vi "DefensePsSkill.vi"(9 "Game in":refnum<class "Game.lvclass">, 10 "Robot":refnum<class "Robot.lvclass">, 11 "DefensePsSkill in":refnum<class "DefensePsSkill.lvclass">) -> (2 "Robot out":refnum<class "Robot.lvclass">, 3 "DefensePsSkill out":refnum<class "DefensePsSkill.lvclass">)   [LabVIEW 2020, in "DefensePsSkill.lvclass"]
uses:
  DefensePsSkill.lvclass
  Robot_class/Robot.lvclass
  Game_class/Game.lvclass
  Utilities_class/Utilities.lvclass
  Game_class/Game.lvclass/Game.ctl
  Object_class/Object.lvclass/Object.ctl
  Ball_class/Ball.lvclass/Ball.ctl
  Team_class/Team.lvclass/Team.ctl
  Robot_class/Robot.lvclass/Robot.ctl
  Game_class/Read BallRef.vi
  Game_class/Read FieldRef.vi
  Game_class/Read EnemyRef.vi
  Team_class/Read RobotRef.vi
  Robot_class/Read orientation.vi
  Object_class/Read x.vi
  Object_class/Read y.vi
  Ball_class/Read v_x.vi
  Ball_class/Read v_y.vi
  Robot_class/Write dest_x.vi
  Robot_class/Write dest_y.vi
  Enemy_class/Enemy.lvclass
  C:/Users/User/Documents/GitHub/SSL_AI/Team_class/Team.lvclass
  Ball_class/Ball.lvclass
  C:/Users/User/Documents/GitHub/SSL_AI/Object_class/Object.lvclass
  Field_class/Field.lvclass
panel:
  out "error out 2":errorcluster
  in  "error in (no error) 2":errorcluster
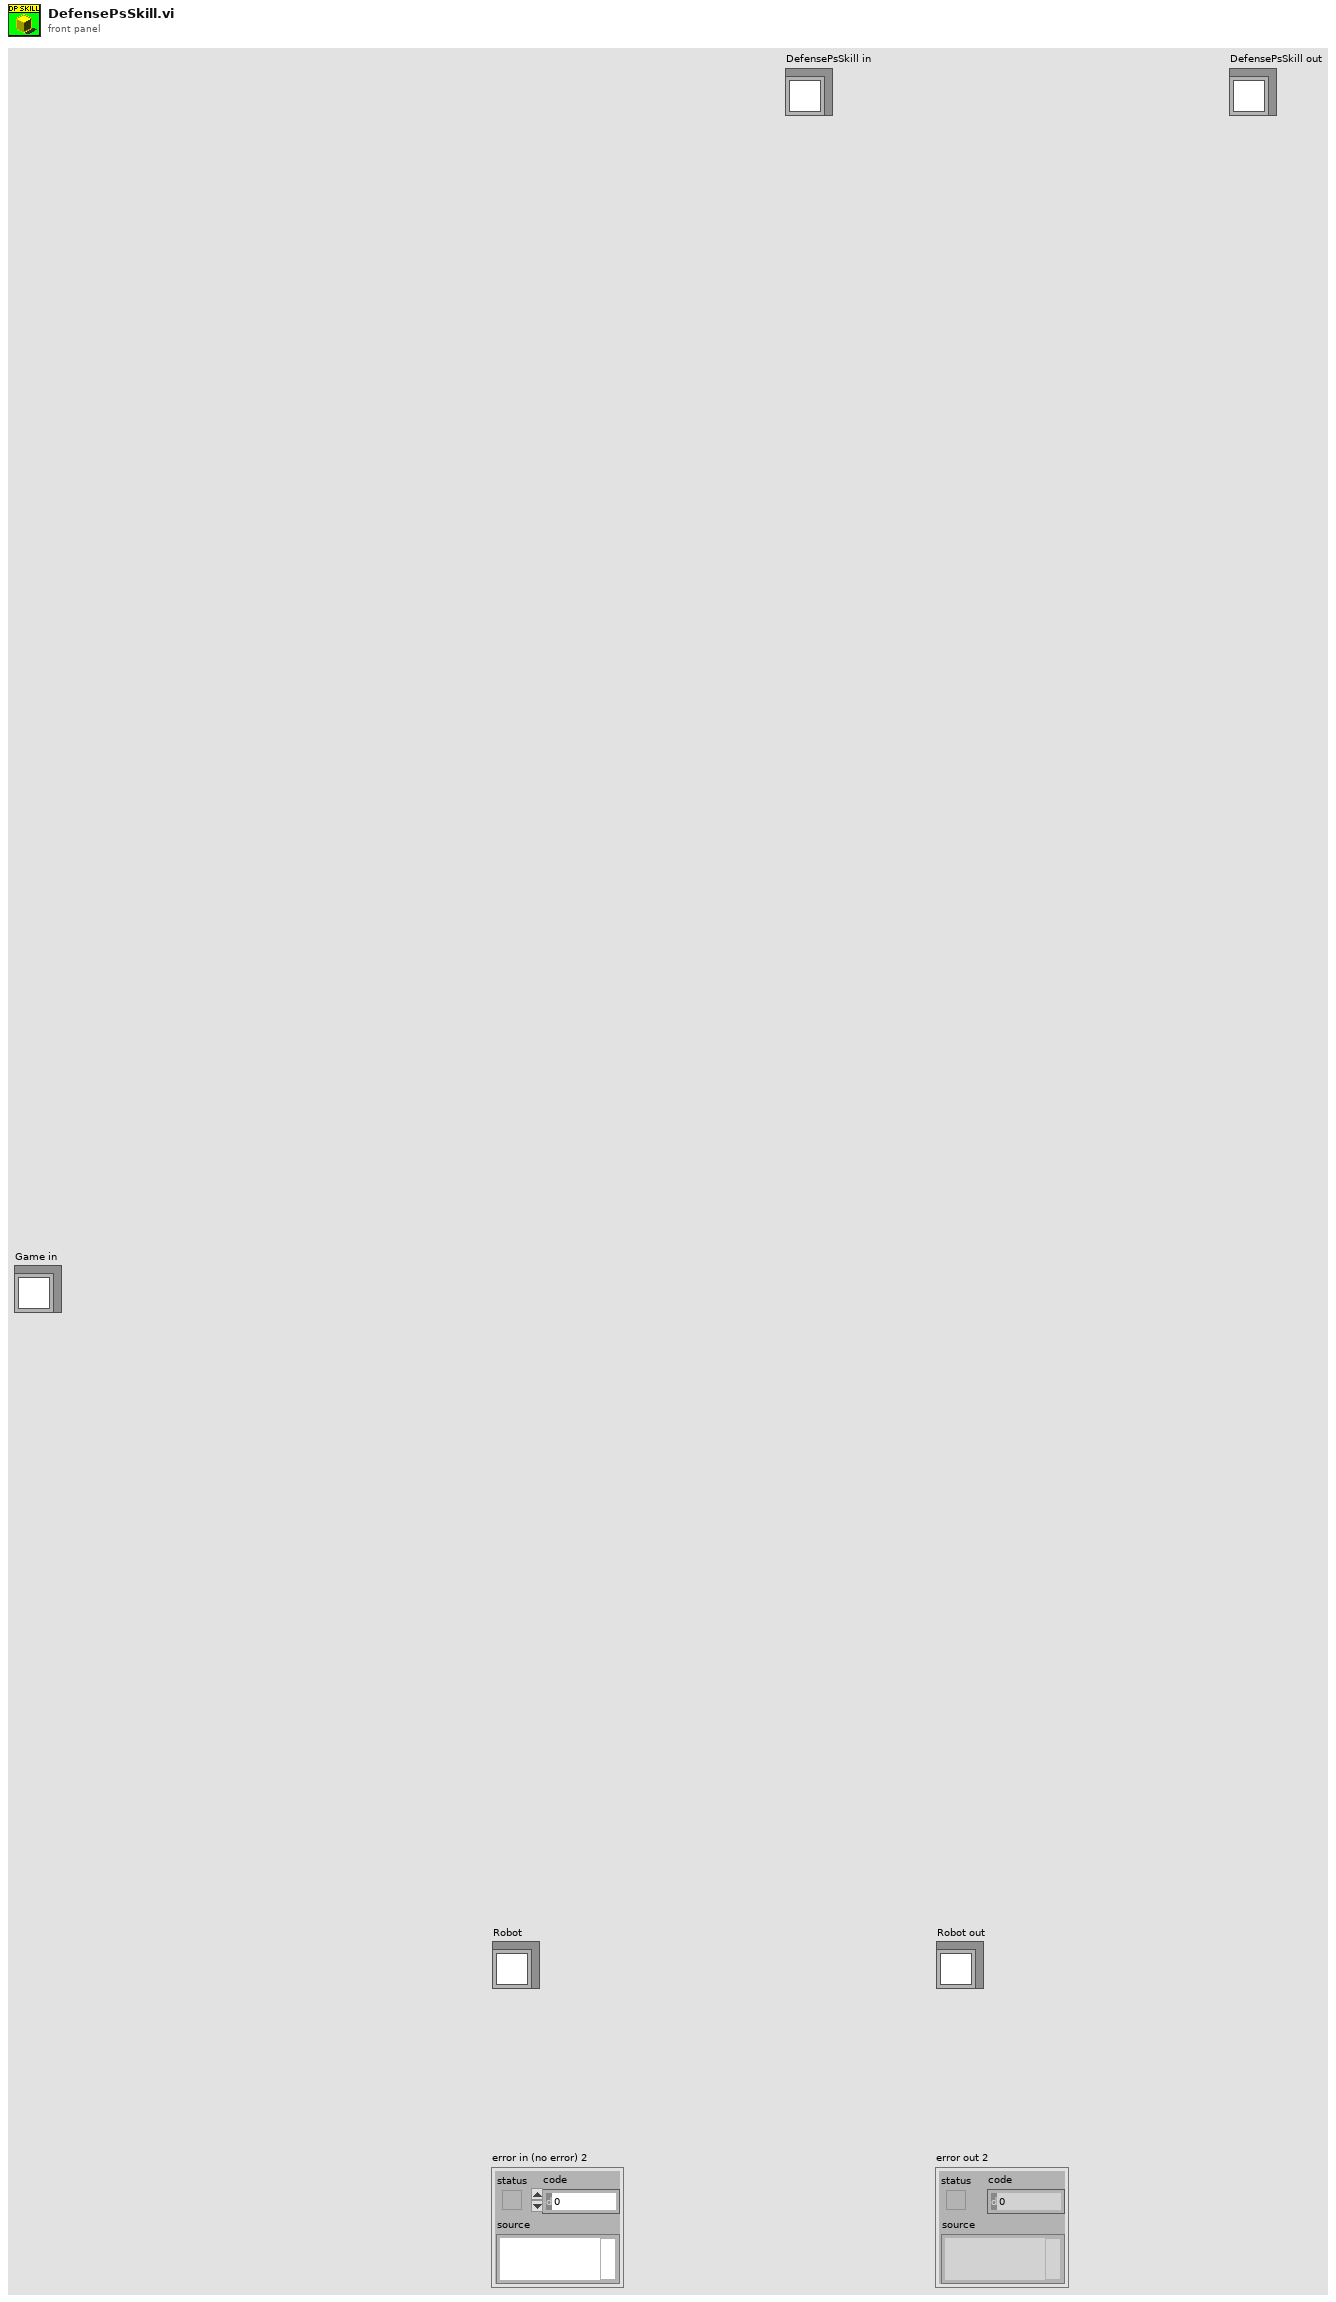
[diagram p1: front panel]
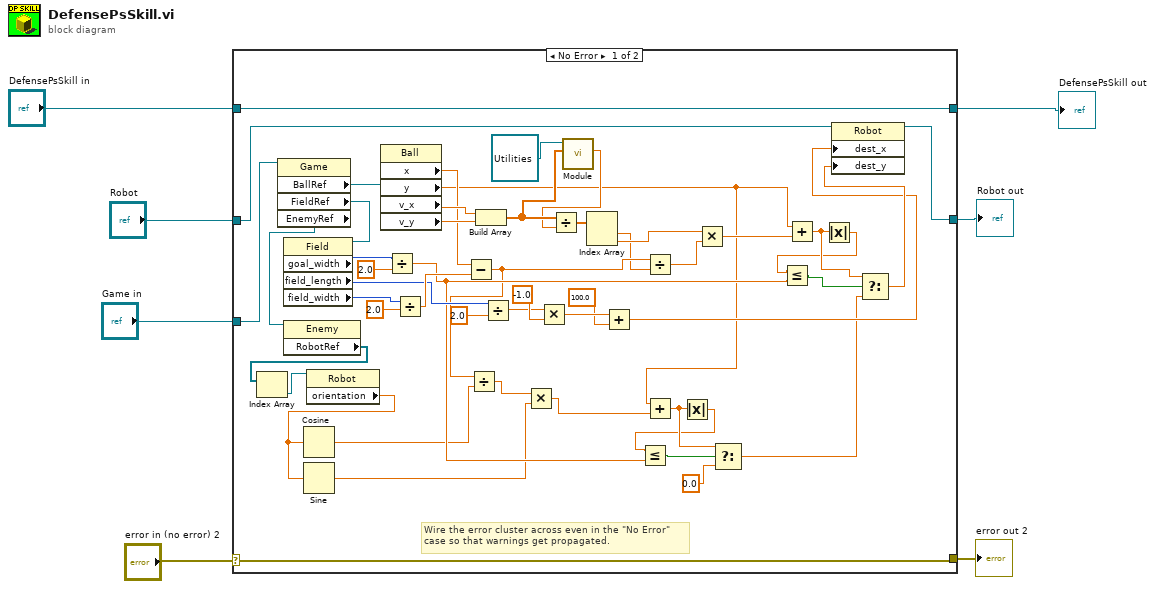
[diagram p0: block diagram]
diagram:
  n1 = case shown="No Error" "error in (no error) 2" {
    selector: "error in (no error) 2" -> [w56 w60]
    tunnel: [w56 w60] -> w6
    tunnel: [w57 w59] -> w2
    tunnel: "DefensePsSkill in" -> [w57 w59]
    tunnel: "Robot" -> [w50 w58]
    tunnel: [w49 w58] -> w4
    tunnel: "Game in" -> [w48 _]
    frame No Error {
      # "Wire the error cluster across even in the \"No Error\"\ncase so that warnings get propagated."
      n2 = property class="Game"(reference=w48) -> ("BallRef"=w53:refnum<class "Ball.lvclass">, "FieldRef"=w54:refnum<class "Field.lvclass">, "EnemyRef"=w28:refnum<class "Enemy.lvclass">)  [unwired: 1 in, 2 out]
      n3 = property class="Field"(reference=w54) -> ("goal_width"=w55:i32, "field_length"=w40:i32, "field_width"=w41:i32)  [unwired: 1 in, 2 out]
      n4 = property class="Enemy"(reference=w28) -> ("RobotRef"=w26:refnum<class "Robot.lvclass">[])  [unwired: 1 in, 2 out]
      n5 = Index Array(array=w26) -> (element=w27:refnum<class "Robot.lvclass">)  [unwired: 1 in]
      n6 = property class="Robot"(reference=w27) -> ("orientation"=w25:dbl)  [unwired: 1 in, 2 out]
      n7 = Cosine(x=w25) -> (cos(x)=w12:dbl)
      n8 = Sine(x=w25) -> (sin(x)=w8:dbl)
      n9 = property class="Ball"(reference=w53) -> ("x"=w45:dbl, "y"=w13:dbl, "v_x"=w47:dbl, "v_y"=w46:dbl)  [unwired: 1 in, 2 out]
      n10 = Divide(x=w55, y=2.0) -> (x/y=w20:dbl)
      n11 = Divide(x=w41, y=2.0) -> (x/y=w44:dbl)
      n12 = Subtract(x=w45, y=w44) -> (x-y=w11:dbl)
      n13 = Divide(x=w11, y=w12) -> (x/y=w9:dbl)
      n14 = Build Array(w47, w46) -> (w33:dbl[])
      n15 = Divide(x=w40, y=2.0) -> (x/y=w38:dbl)
      n16 = Multiply(x=w9, y=w8) -> (x*y=w14:dbl)
      n17 = Multiply(x=w38, y=-1.0) -> (x*y=w37:dbl)
      n18 = call-dynamic "Module.vi"("2D vector"=w33, "Utilities in"=refnum<class "Utilities.lvclass"> refnum) -> ("Modulo"=w32:dbl)  [unwired: 7 in, 2 out]
      n19 = Divide(x=w33, y=w32) -> (x/y=w17:dbl[])
      n20 = Index Array(array=w17) -> (element #1=w10:dbl, element #2=w15:dbl)  [unwired: 2 in]
      n21 = Add(x=w37, y=100.0) -> (x+y=w35:dbl)
      n22 = Divide(x=w11, y=w10) -> (x/y=w16:dbl)
      n23 = Add(x=w13, y=w14) -> (x+y=w24:dbl)
      n24 = Absolute Value(x=w24) -> (abs(x)=w23:dbl)
      n25 = Less Or Equal?(x=w23, y=w20) -> (x <= y?=w22:bool)
      n26 = Multiply(x=w15, y=w16) -> (x*y=w18:dbl)
      n27 = Select(t=w24, s=w22, f=0.0) -> (s? t:f=w19:dbl)
      n28 = Add(x=w13, y=w18) -> (x+y=w31:dbl)
      n29 = Absolute Value(x=w31) -> (abs(x)=w30:dbl)
      n30 = Less Or Equal?(x=w30, y=w20) -> (x <= y?=w29:bool)
      n31 = Select(t=w31, s=w29, f=w19) -> (s? t:f=w42:dbl)
      n32 = property class="Robot"(reference=w50, "dest_x"=w35, "dest_y"=w42) -> (reference out=w49:refnum<class "Robot.lvclass">)  [unwired: 1 in, 1 out]
    }
    frame Error {
    }
  }
  "DefensePsSkill out" <- w2
  "error out 2" <- w6
  "Robot out" <- w4
